vi "WPI_CounterToDigitalSource.vi"   [LabVIEW 2017]
doc: "Converts a digital input, analog trigger output, or digital output to a digital source. Wire the <B>Digital Source</B> output of this VI to VIs that require a digital source, such as the Open VIs on the <B>Counter</B> and <B>Encoder</B> palettes.\n\nThis software is licensed. Open the labview\\readme\\WPI Robotics Library Open Source License.txt file for more information."
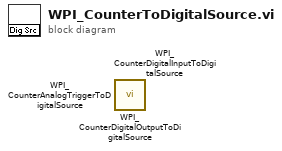
[diagram p0: block diagram]
diagram:
  n1 = call <vilib>:"WPI_CounterDigitalOutputToDigitalSource.vi"() -> ()  [unwired: 7 in, 1 out]
  n2 = call <vilib>:"WPI_CounterDigitalInputToDigitalSource.vi"() -> ()  [unwired: 7 in, 1 out]
  n3 = call <vilib>:"WPI_CounterAnalogTriggerToDigitalSource.vi"() -> ()  [unwired: 7 in, 1 out]
